vi "FTW-Actor-CheckShutdown.vi"(0 "FTW Actor Instance":refnum<class "FTW-Actor-Instance.lvclass">, 11 "error in":errorcluster) -> (4 "FTW Actor Instance out":refnum<class "FTW-Actor-Instance.lvclass">, 6 "Shutdown?":bool, 15 "error out":errorcluster)   [LabVIEW 2015, in "FTW-Actor-Instance.lvclass"]
uses:
  FTW-Actor-Instance.lvclass
  FTW-Actor-Instance.lvclass/FTW-Actor-Instance.ctl
  scheduler/FTW-Scheduler.lvclass
panel:
  # "Inputs"
  # "Outputs"
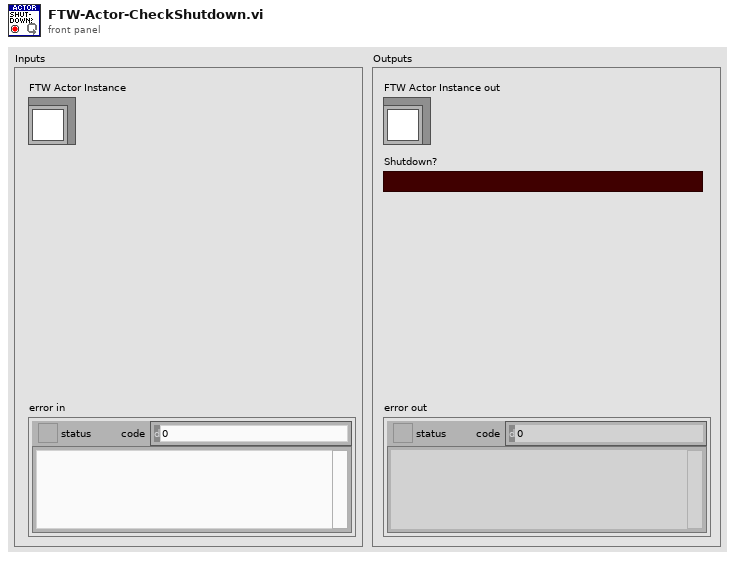
[diagram p1: front panel]
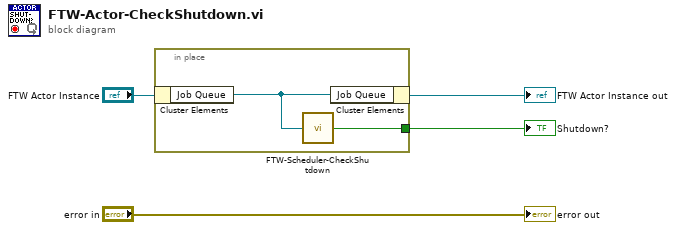
[diagram p0: block diagram]
diagram:
  n1 = in-place {
    in-place-border: [w6] -> w1
    n2 = in-place-cluster #1("FTW Actor Instance") -> ("Job Queue"=w5:refnum<class "FTW-Scheduler.lvclass">)
    n3 = call "FTW-Scheduler-CheckShutdown.vi"("FTW Job Scheduler"=w5) -> ("Shutdown?"=w6:bool)
    n4 = in-place-cluster #1("Job Queue"=w5) -> (→"FTW Actor Instance out":refnum<class "FTW-Actor-Instance.lvclass">)
  }
  "Shutdown?" <- w1
  "error out" <- "error in"
